vi "RSNRPZ Set Scope Auto Resolution.vi"(8 "error in (no error)":errorcluster, 9 "Resolution (3)":i32=3, 10 "Channel (1)":i32=1, 11 "VISA session":refnum<visa-resource-name> caption="VISA resource name") -> (0 "error out":errorcluster, 3 "dup VISA session":refnum<visa-resource-name> caption="VISA resource name")   [LabVIEW 2010]
doc: "This VI defines the number of significant places for linear units and the number of decimal places for logarithmic units which should be free of noise in the measurement result. This setting does not affect the setting of display.\n\nRemote-control command(s):\nSENS:AVER:COUN:AUTO:RES 1 ... 4"
uses:
  rsnrpz_32.dll
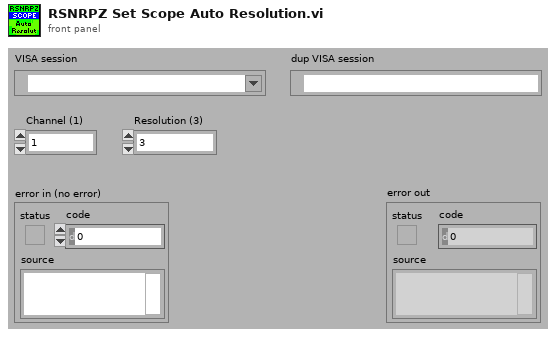
[diagram p1: front panel]
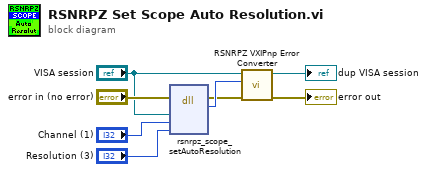
[diagram p0: block diagram]
diagram:
  n1 = dll-call lib="rsnrpz_32.dll" fn="rsnrpz_scope_setAutoResolution"(error in="error in (no error)", "Instrument Handle"="VISA session", "Channel"="Channel (1)", "Resolution"="Resolution (3)") -> (error out=w5:errorcluster, "Status"=w8:i32)  [unwired: 5 in, 1 out]
  n2 = call <instrlib>:"RSNRPZ VXIPnp Error Converter.vi"("error in"=w5, "VXIPnp error code"=w8, "VISA session"="VISA session") -> ("error out"=→"error out":errorcluster, "dup VISA session"=→"dup VISA session":refnum<visa-resource-name>)  [unwired: 7 in]
